vi "Page_Source_Settings_Initialize.vi"(8 "error in (no error)":errorcluster, 9 "ctlReferences":T2, 11 "AB_PackedLibrary in":refnum<class "AB_PackedLibrary.lvclass">) -> (0 "error out":errorcluster, 1 "supportedFunctions":T1, 3 "AB_PackedLibrary out":refnum<class "AB_PackedLibrary.lvclass">)   [LabVIEW 2020, in "AB_PackedLibrary.lvclass"]
uses:
  <vilib>/AppBuilder/AB_Classes/PackedLib/AB_PackedLibrary.lvclass
  <resource>/Framework/Providers/Builds/AppBuilder/AB_UI_Page_Source_Settings_References.ctl
  <resource>/Framework/Providers/Builds/AppBuilder/AB_UI_Page_Source_Settings_supportedFunctions.ctl
  <resource>/Framework/Providers/Common/provcom_StringGlobals.vi
  <vilib>/AppBuilder/AB_Classes/TargetFile/AB_Targetfile.lvclass
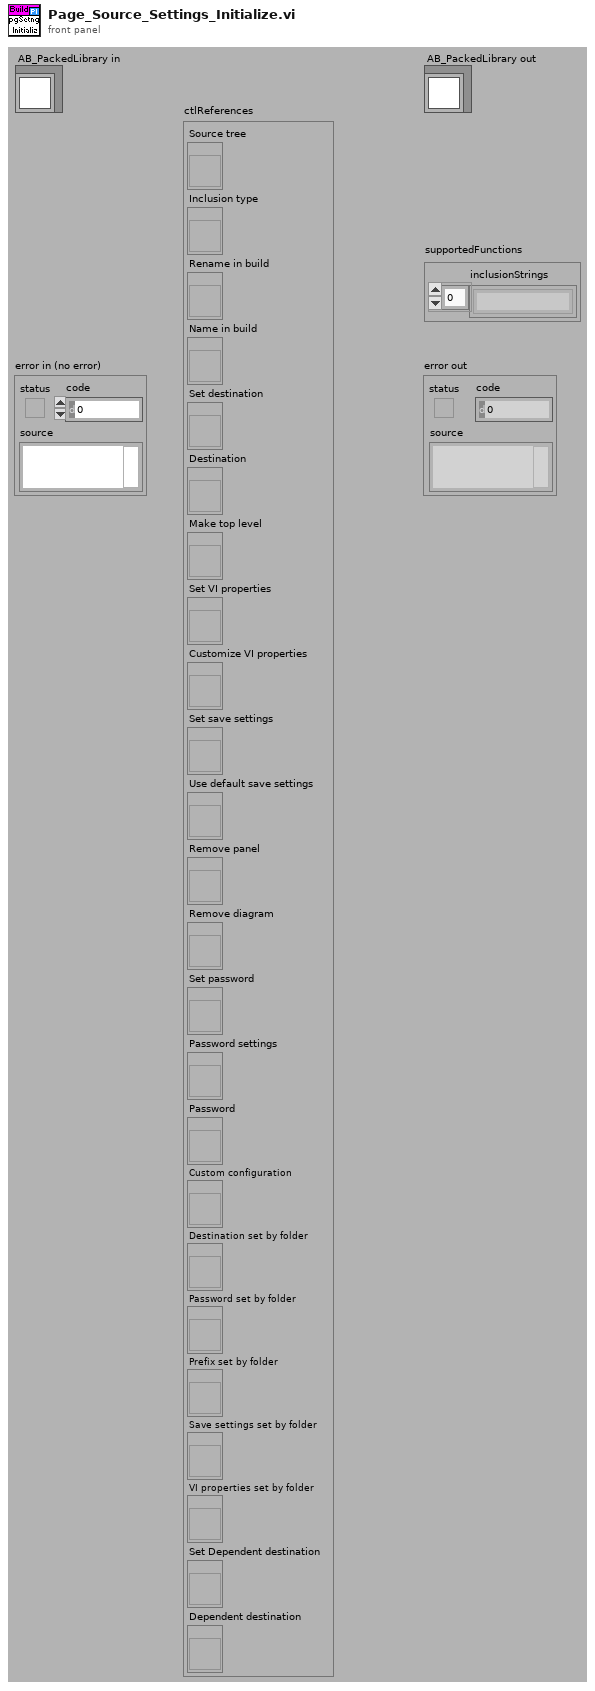
[diagram p1: front panel]
types:
  T1 = typedef "AB_UI_Page_Source_Settings_supportedFunctions.ctl" = cluster{"inclusionStrings":string[]}
  T2 = typedef "AB_UI_Page_Source_Settings_References.ctl" = cluster{"Source tree":refnum<vi>, "Inclusion type":refnum<vi>, "Rename in build":refnum<vi>, "Name in build":refnum<vi>, "Set destination":refnum<vi>, "Destination":refnum<vi>, "Make top level":refnum<vi>, "Set VI properties":refnum<vi>, "Customize VI properties":refnum<vi>, "Set save settings":refnum<vi>, "Use default save settings":refnum<vi>, "Remove panel":refnum<vi>, "Remove diagram":refnum<vi>, "Set password":refnum<vi>, "Password settings":refnum<vi>, "Password":refnum<vi>, "Custom configuration":refnum<vi>, "Destination set by folder":refnum<vi>, "Password set by folder":refnum<vi>, "Prefix set by folder":refnum<vi>, "Save settings set by folder":refnum<vi>, "VI properties set by folder":refnum<vi>, "Set Dependent destination":refnum<vi>, "Dependent destination":refnum<vi>}
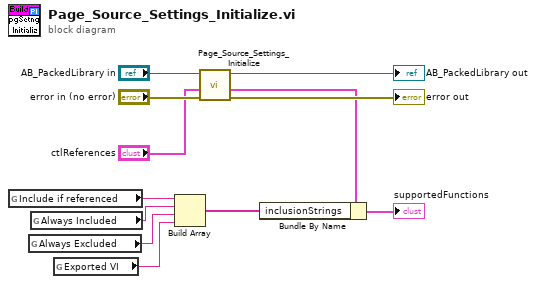
[diagram p0: block diagram]
diagram:
  n1 = global read "provcom_StringGlobals.vi" "Include if referenced"() -> (w5:string)
  n2 = global read "provcom_StringGlobals.vi" "Always Excluded"() -> (w7:string)
  n3 = global read "provcom_StringGlobals.vi" "Always Included"() -> (w6:string)
  n4 = global read "provcom_StringGlobals.vi" "Exported VI"() -> (w4:string)
  n5 = Build Array(w5, w6, w7, w4) -> (w3:string[])
  n6 = call-parent "Page_Source_Settings_Initialize.vi"("error in (no error)"="error in (no error)", "ctlReferences"="ctlReferences", "AB_Build in"="AB_PackedLibrary in") -> ("error out"=→"error out":errorcluster, "supportedFunctions"=w2:T1, "AB_Build out"=→"AB_PackedLibrary out":refnum<class "AB_PackedLibrary.lvclass">)  [unwired: 6 in]
  n7 = Bundle By Name(cluster=w2, "inclusionStrings"=w3) -> (→"supportedFunctions":T1)
